vi "Main.vi"() -> ()   [LabVIEW 2015]
panel:
  out "Version":string
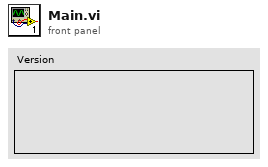
[diagram p1: front panel]
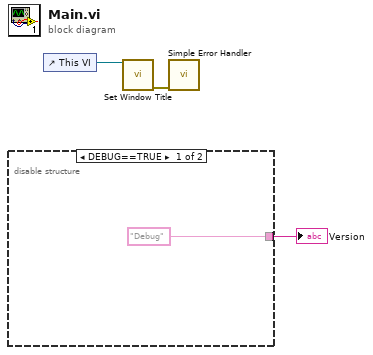
[diagram p0: block diagram]
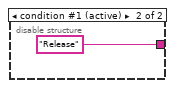
[diagram p2: hidden frame]
diagram:
  n1 = disable-structure shown="DEBUG==TRUE" {
    disable-tunnel: ["Debug" ("Version") "Release" ("Version")] -> w3
    frame condition #0 {
    }
    frame condition #1 (active) {
    }
  }
  "Version" <- w3
  n2 = control-ref of="This VI"() -> (w2:refnum<vi>)
  n3 = call "Set Window Title.vi"("VI in"=w2) -> ("error out"=w1:errorcluster)  [unwired: 14 in]
  n4 = call <vilib>:"Simple Error Handler.vi"("error in (no error)"=w1) -> ()  [unwired: 4 in, 5 out]
